vi "Notify PV Monitoring.vi"(8 "error in (no error)":errorcluster, 11 "CS++DSMonitor in":refnum<class "CS++DSMonitor.lvclass">) -> (0 "error out":errorcluster, 3 "CS++DSMonitor out":refnum<class "CS++DSMonitor.lvclass">)   [LabVIEW 2015, in "CS++DSMonitor.lvlib" / "CS++DSMonitor.lvclass"]
doc: "Notify PV readout."
uses:
  CS++DSMonitor.lvclass
  CS++PVMonitor/CS++PVMonitor.lvclass/CS++PVMonitor.ctl
  CS++DSMonitor.lvclass/CS++DSMonitor.ctl
  <vilib>/ActorFramework/Message Enqueuer/Message Enqueuer.lvclass
  CS++PVMonitor Messages/CS++PVUpdate Msg/CS++PVUpdate Msg.lvclass
  CS++PVMonitor/CS++PVMonitor.lvclass
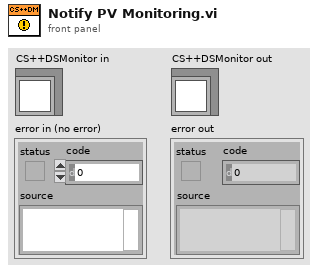
[diagram p1: front panel]
types:
  T1 = cluster{"PV URL":string, "Observers":cluster{"Enqueuer":refnum<class "Message Enqueuer.lvclass">, "CS++PVUpdate Msg":refnum<class "CS++PVUpdate Msg.lvclass">}[]}[]
  T2 = cluster{"DS Refnums":refnum<k13>[], "PV Connections":cluster{"PV URL":string, "Observers":cluster{"Enqueuer":refnum<class "Message Enqueuer.lvclass">, "CS++PVUpdate Msg":refnum<class "CS++PVUpdate Msg.lvclass">}[]}[]}
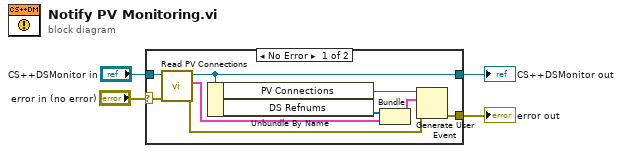
[diagram p0: block diagram]
diagram:
  n1 = case shown="No Error" "error in (no error)" {
    selector: "error in (no error)" -> [w12 w14]
    tunnel: "CS++DSMonitor in" -> [w13 w15]
    tunnel: [w9 w15] -> w2
    tunnel: [w5 w14] -> w1
    frame No Error {
      n2 = call "Read PV Connections.vi"("error in (no error)"=w12, "CS++PVMonitor in"=w13) -> ("error out"=w6:errorcluster, "PV Connections"=w10:T1, "CS++PVMonitor out"=w9:refnum<class "CS++DSMonitor.lvclass">)  [unwired: 7 in]
      n3 = Unbundle By Name(w9) -> ("PV Connections"=w8:refnum<user-event>, "DS Refnums"=w11:refnum<k13>[])
      n4 = Bundle("DS Refnums"=w11, "PV Connections"=w10) -> (w7:T2)  [unwired: 1 in]
      n5 = Generate User Event(user event=w8, event data cluster=w7, error in=w6) -> (error out=w5:errorcluster)  [unwired: 1 in, 1 out]
    }
    frame Error {
    }
  }
  "error out" <- w1
  "CS++DSMonitor out" <- w2
